vi "Wait for Delay Position.vi"(6 "Timeout":u32=10000, 8 "error in (no error)":errorcluster, 9 "Range":dbl=0.001, 10 "Position":dbl, 11 "Axis":i32) -> (0 "error out":errorcluster)   [LabVIEW 2019, in "Acquisition Example.lvlib"]
uses:
  Acquisition Example.lvlib
  <vilib>/Utility/error.llb/Error Cluster From Error Code.vi
  <vilib>/ErrorRing/Error Ring.xnode
  ESP301/ESP301.lvlib
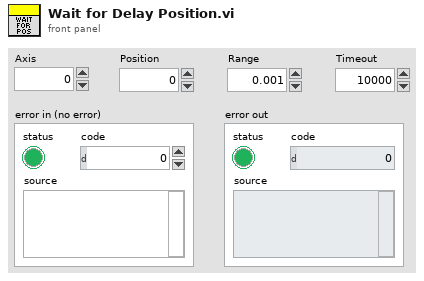
[diagram p1: front panel]
types:
  T1 = typedef "ESP301.lvlib/Get Position (Reply Payload)--cluster.ctl" = cluster{"Position":dbl, "Get Position_error":errorcluster, "Axis":i32}
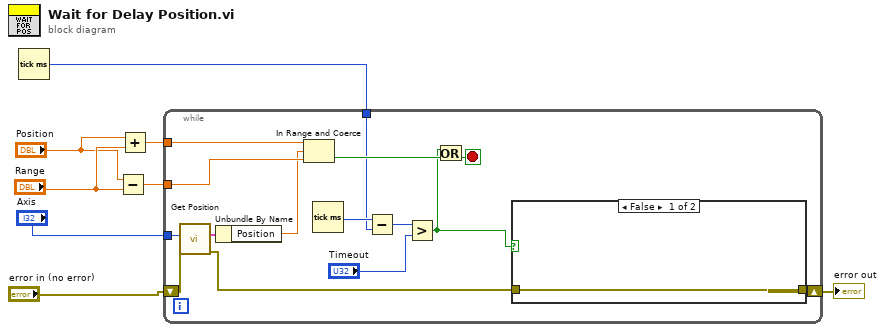
[diagram p0: block diagram]
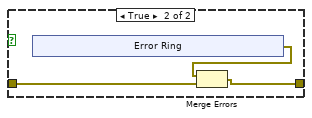
[diagram p2: hidden frame]
diagram:
  n1 = Tick Count (ms)() -> (millisecond timer value=w1:u32)
  n2 = Subtract(x="Position", y="Range") -> (x-y=w5:dbl)
  n3 = Add(x="Position", y="Range") -> (x+y=w2:dbl)
  n4 = while {
    tunnel: "Axis" -> [w23]
    tunnel: w5 -> [w21]
    tunnel: w2 -> [w20]
    shift-right: [w12] -> w7
    shift-left: "error in (no error)" -> [w22]
    tunnel: w1 -> [w16]
    stop <- w13 stop-if-true
    n5 = call "Get Position.vi"("error in (no error)"=w22, "Axis"=w23) -> ("error out"=w11:errorcluster, "Reply Payload"=w9:T1)  [unwired: 7 in, 1 out]
    n6 = Unbundle By Name(w9) -> ("Position"=w19:dbl)
    n7 = In Range and Coerce(upper limit=w20, x=w19, lower limit=w21) -> (In Range?=w18:bool)  [unwired: 1 out]
    n8 = Tick Count (ms)() -> (millisecond timer value=w17:u32)
    n9 = Subtract(x=w17, y=w16) -> (x-y=w15:u32)
    n10 = Greater?(x=w15, y="Timeout") -> (0:w10:bool)
    n11 = Or(x=w10, y=w18) -> (x .or. y?=w13:bool)
    n12 = case shown="False" w10 {
      tunnel: [w24 w26] -> w12
      tunnel: w11 -> [w24 w27]
      frame False {
      }
      frame True {
        n13 = xnode "Error Ring"() -> ("error out"=w25:errorcluster)
        n14 = Merge Errors(w25, w27) -> (w26:errorcluster)
      }
    }
  }
  "error out" <- w7
